vi "mod_Get Kaiser Filter Parameters.vi"(4 "ws":dbl=0.6, 6 "wp":dbl=0.4, 10 "len":i32=12, 11 "I":i32=128) -> (2 "Rs":dbl=8.0, 3 "beta":dbl)   [LabVIEW 2020, in "niAMT.lvlib"]
uses:
  <vilib>/addons/Modulation/niAMT.lvlib
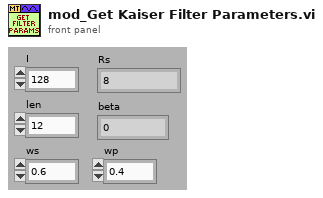
[diagram p1: front panel]
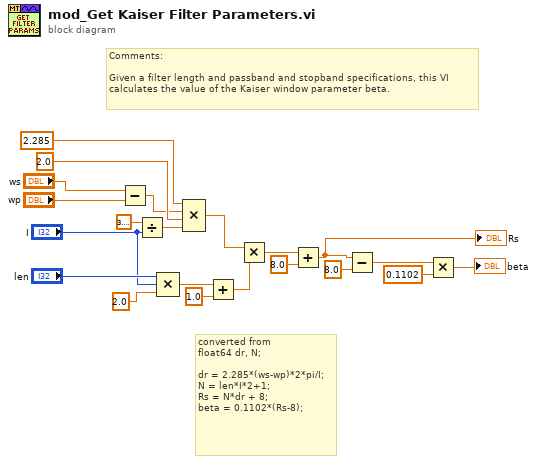
[diagram p0: block diagram]
diagram:
  # "converted from\nfloat64 dr, N;\n\ndr = 2.285*(ws-wp)*2*pi/I;\nN = len*I*2+1;\nRs = N*dr + 8;\nbeta = 0.1102*(Rs-8);"
  # "Comments: \n\nGiven a filter length and passband and stopband specifications, this VI\ncalculates the value of the Kaiser window parameter beta."
  n1 = Subtract(x="ws", y="wp") -> (x-y=w19:dbl)
  n2 = Divide(x=3.141592653589793, y="I") -> (x/y=w21:dbl)
  n3 = Compound Arithmetic op=MULTIPLY("len", "I", 2.0 ("value")) -> (w15:dbl)
  n4 = Compound Arithmetic op=MULTIPLY(2.285 ("value"), w19, 2.0 ("value"), w21) -> (w13:dbl)
  n5 = Add(x=w15, y=1.0) -> (x+y=w7:dbl)
  n6 = Multiply(x=w13, y=w7) -> (x*y=w12:dbl)
  n7 = Add(x=w12, y=8.0) -> (x+y=w5:dbl)
  "Rs" <- w5
  n8 = Subtract(x=w5, y=8.0) -> (x-y=w9:dbl)
  n9 = Multiply(x=w9, y=0.1102) -> (x*y=→"beta":dbl)
